vi "Front Panel Control Variables.vi"() -> ()   [LabVIEW 2016, in "Shared resources RT.lvlib"]
uses:
  Shared resources RT.lvlib
panel:
  in  "VEL":u16=850
  in  "Send vel":bool
  in  "Reset Errors":bool
  in  "resetPID":bool
  in  "UseGPS":bool
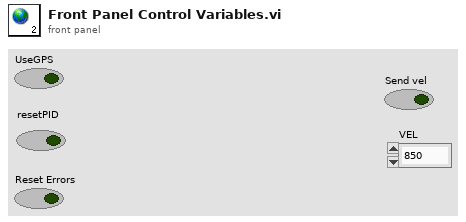
[diagram p1: front panel]
diagram:
